vi "AWG Get Capabilities.vi"(8 "error in (no error)":errorcluster, 11 "awg session":T1) -> (0 "error out":errorcluster, 2 "has cfg panel?":bool, 3 "awg session out":T1)   [LabVIEW 2020, in "AWG.lvlib"]
doc: "Get selected AWG capabilities."
uses:
  AWG.lvlib
  AWG Session.ctl
  AWG Type.ctl
  CMI Clock Divider v2/CMI ckd2 Session.ctl
  CMI Clock Divider v2/CMI ckd2 Source Mode.ctl
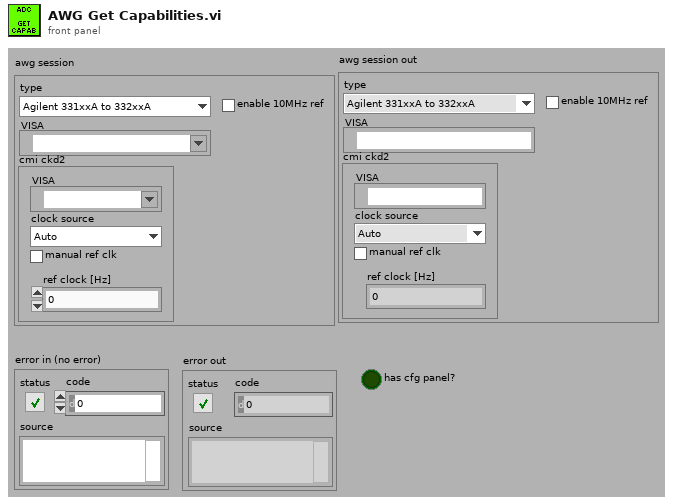
[diagram p1: front panel]
types:
  T1 = typedef "AWG.lvlib/AWG Session.ctl" = cluster{"type":T2, "VISA":refnum<visa-resource-name>, "enable 10MHz ref":bool, "cmi ckd2":T3}
  T2 = typedef "AWG.lvlib/AWG Type.ctl" = enum16{"Agilent 331xxA to 332xxA", "Agilent 335xxA to 336xxA", "Tektronix AFG3101C", "CMI Clock Divider v2", "dummy"}
  T3 = typedef "AWG.lvlib/CMI ckd2 Session.ctl" = cluster{"VISA":refnum<visa-resource-name>, "clock source":T4, "manual ref clk":bool, "ref clock [Hz]":dbl}
  T4 = typedef "AWG.lvlib/CMI ckd2 Source Mode.ctl" = enum16{"Auto", "LF clock", "HF clock", "Internal"}
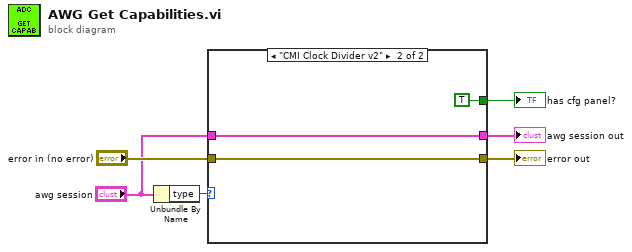
[diagram p0: block diagram]
diagram:
  n1 = Unbundle By Name("awg session") -> ("type"=w4:T2)
  n2 = case shown="\"CMI Clock Divider v2\"" w4 {
    tunnel: "error in (no error)" -> [w7 w11]
    tunnel: [w7 w11] -> w5
    tunnel: "awg session" -> [w8 w10]
    tunnel: [w8 w10] -> w2
    tunnel: [_ TRUE] -> w1
    frame Default {
    }
    frame "CMI Clock Divider v2" {
    }
  }
  "error out" <- w5
  "awg session out" <- w2
  "has cfg panel?" <- w1
